vi "Digital Read Multiple Channels.vi"(8 "error in (no error)":errorcluster, 10 "Array":i32[](array[numeric]), 11 "NI-DAQ in":refnum<class "NI-DAQ.lvclass">) -> (0 "error out":errorcluster, 2 "subarray":bool[](array[boolean]), 3 "NI-DAQ out":refnum<class "NI-DAQ.lvclass">)   [LabVIEW 2021, in "NI-DAQ.lvclass"]
uses:
  NI-DAQ.lvclass
  NI-DAQ.lvclass/NI-DAQ.ctl
  <vilib>/Utility/file.llb/Read Delimited Spreadsheet (string).vi
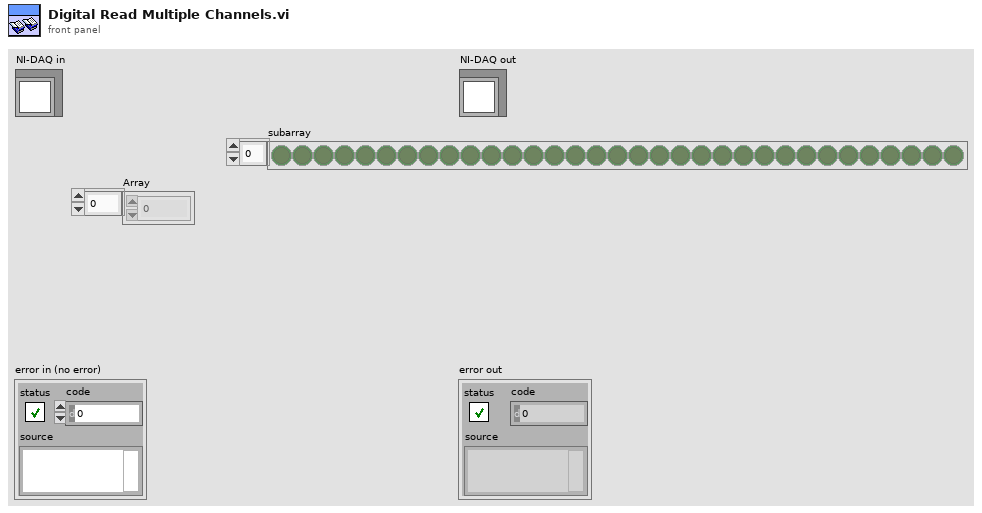
[diagram p1: front panel]
types:
  T1 = typedef "File Paths.ctl" = cluster{"Glue Pattern Folder":path, "Carrier Tray Folder":path, "Pick Up Tool Fixture Folder":path, "Components Folder":path, "Bellows Tool Offset.txt":path, "Pick Up Tool Offset.txt":path, "Dispense Tip Offset.txt":path, "Log Files":path, "Gantry Assembly Map.txt":path, "Syringe and offset map.txt":path, "Controllers Folder":path, "Local dbase config":path}
  T2 = typedef "I-O.lvclass/Pin Map.ctl" = cluster{"Region Valves":i32[], "Extra Valves":dbl[][][], "Tool Primary Valve":i32, "Tool Secondary Valve":i32, "Region Sensors":i32[], "Extra Sensors":dbl[][][], "Tool Primary Sensor":dbl, "Tool Secondary Sensor":dbl, "Compression Sensor":dbl, "5V":i32, "Dispenser Sensor":dbl}
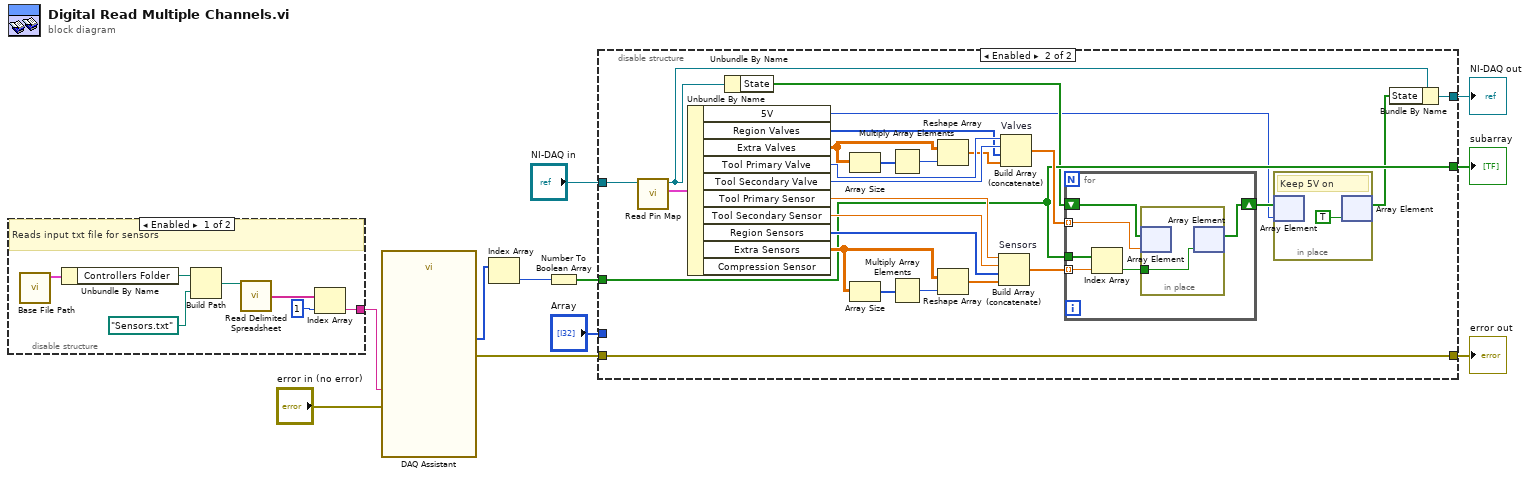
[diagram p0: block diagram]
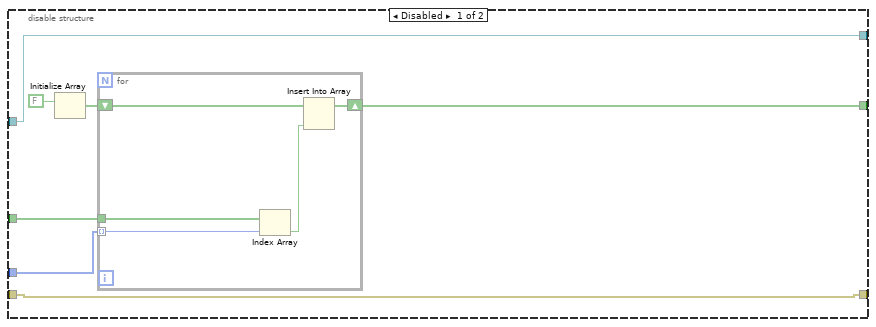
[diagram p3: hidden frame]
diagram:
  n1 = disable-structure shown="Enabled" {
    disable-tunnel: [w12 _] -> w1
    frame Enabled {
      # "Reads input txt file for sensors"
      n2 = call "Base File Path.vi"() -> ("Paths Out"=w18:T1)  [unwired: 11 in]
      n3 = Unbundle By Name(w18) -> ("Controllers Folder"=w17:path)
      n4 = Build Path(base path=w17, name or relative path=path "Sensors.txt") -> (appended path=w15:path)
      n5 = call-poly <vilib>:"Read Delimited Spreadsheet.vi"("file path (dialog if empty)"=w15) -> ("first row"=w14:string[])  [unwired: 9 in, 5 out]
      n6 = Index Array(array=w14, index=1 ("dimension size")) -> (element=w12:string)
    }
    frame Disabled {
    }
  }
  n7 = call "DAQ Assistant"("error in"="error in (no error)", "device name"=w1) -> ("data"=w2:u32[], "error out"=w3:errorcluster)  [unwired: 15 in, 1 out]
  n8 = Index Array(array=w2) -> (element=w11:u32)  [unwired: 1 in]
  n9 = Number To Boolean Array(number=w11) -> (Boolean array=w10:bool[])
  n10 = disable-structure shown="Enabled" {
    disable-tunnel: w10 -> [w25 w35]
    disable-tunnel: "Array" -> [w24 _]
    disable-tunnel: [w21 w35] -> w8
    disable-tunnel: [w20 w56] -> w6
    disable-tunnel: "NI-DAQ in" -> [w20 w54]
    disable-tunnel: [w19 w55] -> w4
    disable-tunnel: w3 -> [w19 w55]
    frame Disabled {
      n11 = Initialize Array(FALSE) -> (w23:bool[])  [unwired: 1 in]
      n12 = for {
        tunnel: w25 -> [w30]
        tunnel: w24 -> [w29] mode=indexing
        shift-right: [w28] -> w21
        shift-left: w23 -> [w27]
        n13 = Index Array(array=w30, index=w29) -> (element=w26:bool)
        n14 = Insert Into Array(array=w27, new element=w26) -> (w28:bool[])  [unwired: 1 in]
      }
    }
    frame Enabled {
      n15 = call-dynamic "Read Pin Map.vi"("NI-DAQ in"=w54) -> ("Pin Map"=w53:T2, "NI-DAQ out"=w52:refnum<class "NI-DAQ.lvclass">)  [unwired: 8 in, 1 out]
      n16 = Unbundle By Name(w53) -> ("5V"=w32:i32, "Region Valves"=w49:i32[], "Extra Valves"=w46:dbl[][][], "Tool Primary Valve"=w51:i32, "Tool Secondary Valve"=w50:i32, "Tool Primary Sensor"=w42:dbl, "Tool Secondary Sensor"=w41:dbl, "Region Sensors"=w40:i32[], "Extra Sensors"=w39:dbl[][][])  [unwired: 1 out]
      n17 = Unbundle By Name(w52) -> ("State"=w34:bool[])
      n18 = Array Size(array=w46) -> (size(s)=w48:i32[])
      n19 = Array Size(array=w39) -> (size(s)=w44:i32[])
      n20 = Multiply Array Elements(1:w48) -> (0:w47:i32)
      n21 = Multiply Array Elements(1:w44) -> (0:w43:i32)
      n22 = Reshape Array(w46, w47) -> (w45:dbl[])
      n23 = Reshape Array(w39, w43) -> (w38:dbl[])
      n24 = Build Array (concatenate) "Sensors"(w42, w41, w40, w38) -> (w36:dbl[])
      n25 = Build Array (concatenate) "Valves"(w51, w50, w49, w45) -> (w37:dbl[])
      n26 = for {
        tunnel: w36 -> [w58] mode=indexing
        tunnel: w35 -> [w62]
        shift-right: [w60] -> w33
        shift-left: w34 -> [w61]
        tunnel: w37 -> [w57] mode=indexing
        n27 = Index Array(array=w62, index=w58) -> (element=w59:bool)
        n28 = in-place {
          in-place-border: w59 -> [w63]
          n29 = in-place-array #1(w61, w57) -> ()  [unwired: 1 out]
          n30 = in-place-array #1(w63) -> (w60:bool[])  [unwired: 1 out]
        }
      }
      n31 = in-place {
        # "Keep 5V on"
        n32 = in-place-array #2(w33, w32) -> ()  [unwired: 1 out]
        n33 = in-place-array #2(TRUE ("element")) -> (w31:bool[])  [unwired: 1 out]
      }
      n34 = Bundle By Name(cluster=w52, "State"=w31) -> (w56:refnum<class "NI-DAQ.lvclass">)
    }
  }
  "error out" <- w4
  "NI-DAQ out" <- w6
  "subarray" <- w8
